vi "Get Request example.vi"(8 "error in (no error)":errorcluster, 10 "Authentication Info":T3={"Client ID"="", "Client Secret"="", "Redirect URI"="", "Token Endpoint"="https://app.asana.com/-/oauth_token", "Scope"=""}, 11 "Asana in":refnum<class "Asana.lvclass">) -> (0 "error out":errorcluster, 2 "Tasks":T1(array[cluster]), 3 "Asana out":refnum<class "Asana.lvclass">)   [LabVIEW 2016, in "Asana.lvclass"]
uses:
  Asana.lvclass
panel:
  in  "Team":T2(ring)
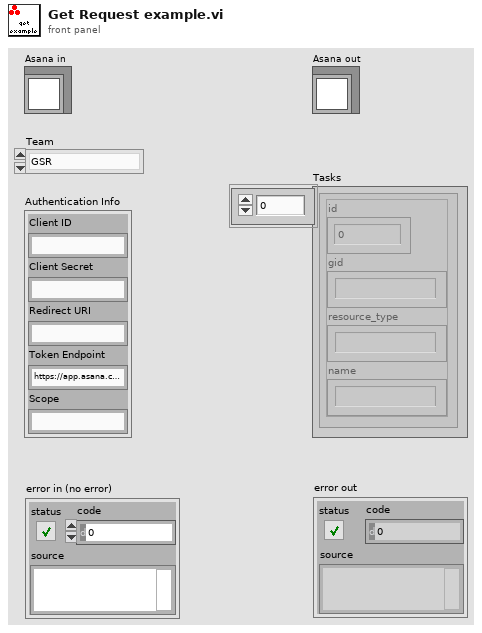
[diagram p1: front panel]
types:
  T1 = cluster{"id":i32, "gid":string, "resource_type":string, "name":string}[]
  T2 = enum16{"GSR", "Research Projects", "Undergrads", "Researchers", "Hardware", "Software", "LevyLab", "Samples", "Manuscripts", "AoT", "WorkStudy"}
  T3 = cluster{"Client ID":string, "Client Secret":string, "Redirect URI":string, "Token Endpoint":string, "Scope":string}
  T4 = cluster{"id":i32, "gid":string, "name":string, "resource_type":string}[]
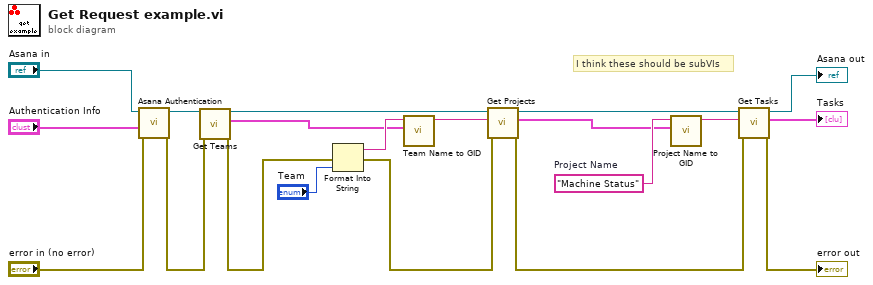
[diagram p0: block diagram]
diagram:
  w10 = "Machine Status"  # Project Name
  # "I think these should be subVIs"
  n1 = call "Asana Authentication.vi"("error in (no error)"="error in (no error)", "Authentication Info"="Authentication Info", "Asana in"="Asana in") -> ("error out"=w6:errorcluster, "Asana out"=w18:refnum<class "Asana.lvclass">)  [unwired: 6 in, 1 out]
  n2 = call "Get Teams.vi"("error in (no error)"=w6, "Asana in"=w18) -> ("error out"=w2:errorcluster, "Teams out"=w7:T4, "Asana out"=w16:refnum<class "Asana.lvclass">)  [unwired: 7 in]
  n3 = Format Into String(error in=w2, "Team") -> (resulting string=w9:string, error out=w1:errorcluster)  [unwired: 2 in]
  n4 = call "Team Name to GID.vi"("Teams in"=w7, "Team Name"=w9) -> ("Team gid"=w17:string)  [unwired: 9 in]
  n5 = call "Get Projects.vi"("error in (no error)"=w1, "Team GID"=w17, "Asana in"=w16) -> ("error out"=w4:errorcluster, "Projects out"=w8:T4, "Asana out"=w14:refnum<class "Asana.lvclass">)  [unwired: 6 in]
  n6 = call "Project Name to GID.vi"("Projects in"=w8, "Name"=w10) -> ("gid"=w15:string)  [unwired: 9 in]
  n7 = call "Get Tasks.vi"("error in (no error)"=w4, "Project GID"=w15, "Asana in"=w14) -> ("error out"=→"error out":errorcluster, "Tasks Out"=→"Tasks":T1, "Asana out"=→"Asana out":refnum<class "Asana.lvclass">)  [unwired: 6 in]
